vi "Date File Name 2012 NIVerified.vi"(9 "Data Count":i32, 10 "Folder to save file to":path=path "C:/Users/Frederic Schmitt/Desktop/GE/Sciospec Bioimpedance - Sinan/Sciospec ISX3v2/Data from LabVIEW") -> (2 "New file path":path)   [LabVIEW 2012]
panel:
  # "Overview: This example VI enables saved files to include the date and time in its filename. \nRequirements: LabVIEW Base Development System 2012 (or compatible)\nInstructions:\n1.\tSet the file path for the files to be saved\n3.\tRun the program"
  # "Set File Name to Current Date/Time"
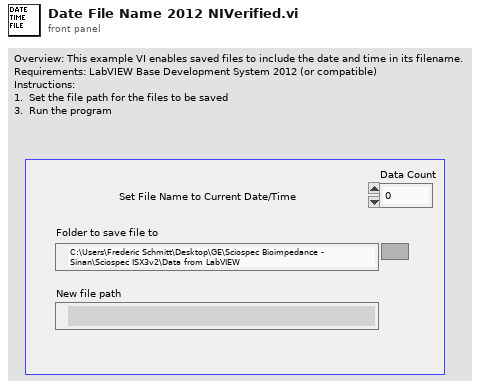
[diagram p1: front panel]
types:
  T1 = enum16{"open", "replace", "create", "open or create", "replace or create", "replace or create with confirmation"}
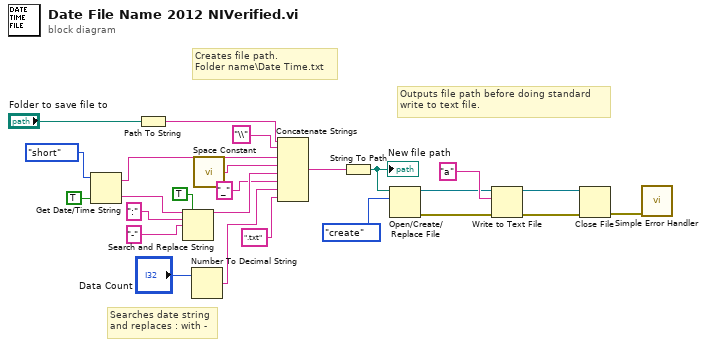
[diagram p0: block diagram]
diagram:
  # "Searches date string\nand replaces : with -"
  # "Creates file path.\nFolder name\\Date Time.txt"
  # "Outputs file path before doing standard\nwrite to text file."
  n1 = Get Date/Time String(date format (0)=enum16{"short", "long", "abbreviated"}."short", want seconds? (F)=TRUE) -> (date string=w7:string, time string=w23:string)  [unwired: 1 in]
  n2 = Path To String(path="Folder to save file to") -> (string=w18:string)
  n3 = Search and Replace String(replace all?=TRUE ("replace all? (F)"), input string=w23, search string=":" ("replace string (\"\")"), replace string="-" ("replace string (\"\")")) -> (result string=w8:string)  [unwired: 4 in, 3 out]
  n4 = Number To Decimal String(number="Data Count") -> (decimal integer string=w5:string)  [unwired: 1 in]
  n5 = call <vilib>:"Space Constant.vi"() -> ("String"=w4:string)
  n6 = Concatenate Strings "Concatenate Strings"(w18, "\\" ("string"), w7, w4, w8, "_" ("string"), w5, ".txt" ("string")) -> (w19:string)
  n7 = String To Path(string=w19) -> (path=w16:path)
  "New file path" <- w16
  n8 = Open/Create/Replace File(file path (use dialog)=w16, operation (0:open)=T1."create") -> (refnum out=w12:refnum<file>, error out=w14:errorcluster)  [unwired: 4 in, 1 out]
  n9 = Write to Text File(file (use dialog)=w12, text="a", error in=w14) -> (refnum out=w10:refnum<file>, error out=w11:errorcluster)  [unwired: 1 in, 1 out]
  n10 = Close File(refnum=w10, error in=w11) -> (error out=w9:errorcluster)  [unwired: 1 out]
  n11 = call <vilib>:"Simple Error Handler.vi"("error in (no error)"=w9) -> ()  [unwired: 4 in, 5 out]
